vi "Main_SubVI_Pulse to Position.vi"(8 "Error In":errorcluster, 10 "Pulse":i32, 11 "Axis Number":T1=1 items=["X"=1, "Y"=2, "Z"=3, "Rotation"=4]) -> (0 "Error Out":errorcluster, 3 "Postion":dbl)   [LabVIEW 2015]
uses:
  Control/Control_Axis Number.ctl
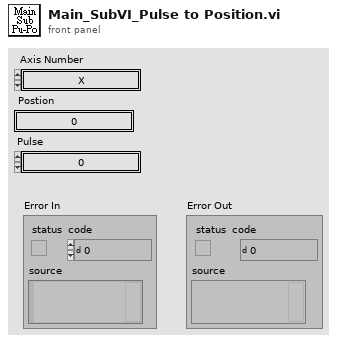
[diagram p1: front panel]
types:
  T1 = typedef "Control_Axis Number.ctl" = u16
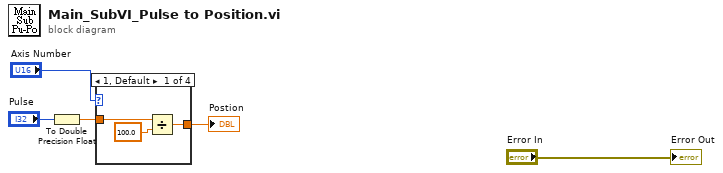
[diagram p0: block diagram]
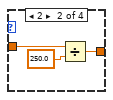
[diagram p2: hidden frame]
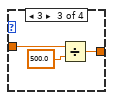
[diagram p3: hidden frame]
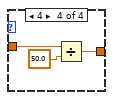
[diagram p4: hidden frame]
diagram:
  n1 = To Double Precision Float(number="Pulse") -> (double precision float=w5:dbl)
  n2 = case shown="1, Default" "Axis Number" {
    tunnel: w5 -> [w8 w11 w14 w17]
    tunnel: [w6 w9 w12 w15] -> w2
    frame 1, Default {
      n3 = Divide(x=w8, y=100.0) -> (x/y=w6:dbl)
    }
    frame 2 {
      n4 = Divide(x=w11, y=250.0) -> (x/y=w9:dbl)
    }
    frame 3 {
      n5 = Divide(x=w14, y=500.0) -> (x/y=w12:dbl)
    }
    frame 4 {
      n6 = Divide(x=w17, y=50.0) -> (x/y=w15:dbl)
    }
  }
  "Postion" <- w2
  "Error Out" <- "Error In"
